vi "Adaptive Parameter 32f.vi"(8 "Error In":errorcluster, 10 "Dynamic Anisotropic Filter Parameters":T1={"Kappa Min"=0.5, "Kappa Max"=10.0, "Time Step"=0.1, "Total Time"=2.0}, 11 "Anisotropic Filter Object":T2={"Device In"=0, "Convolution Object"={"Device In"=0, "Program Handle"=0, "Kernel Memory Object"={"Device ID"=0, "Memeroy ID"=0, "Dimension"={"Depth"=0, "Height"=0, "Width"=0}, "Memory Type"=enum."32f"}, "Convolved Memory Object"={"Device ID"=0, "Memeroy ID"=0, "Dimension"={"Depth"=0, "Height"=0, "Width"=0}, "Memory Type"=enum."32f"}}, "Imag Kernel"=[], "Real Kernel"=[], "Convolved Buffer"={"Device ID"=0, "Memeroy ID"=0, "Dimension"={"Depth"=0, "Height"=0, "Width"=0}, "Memory Type"=enum."32f"}, "Program Handle"=0, "Ansiotropic Filter Parameters"={"Time Step"=0.0, "Total Time"=0.5, "Std. Deviation"=0.0, "Gaussian Filter X Size"=1, "Gaussian Filter Y Size"=1, "Gaussian Filter Z Size"=1}, "Raw Data"={"Device ID"=0, "Memeroy ID"=0, "Dimension"={"Depth"=0, "Height"=0, "Width"=0}, "Memory Type"=enum."32f"}, "Buffer 3"={"Device ID"=0, "Memeroy ID"=0, "Dimension"={"Depth"=0, "Height"=0, "Width"=0}, "Memory Type"=enum."32f"}, "Dimensions"={"Depth"=1, "Height"=1, "Width"=1}} {"Dimensions"."Width" min=1; "Dimensions"."Height" min=1; "Dimensions"."Depth" min=1; "Buffer 3"."Dimension"."Width" min=1; "Buffer 3"."Dimension"."Height" min=1; "Buffer 3"."Dimension"."Depth" min=1; "Raw Data"."Dimension"."Width" min=1; "Raw Data"."Dimension"."Height" min=1; "Raw Data"."Dimension"."Depth" min=1; "Ansiotropic Filter Parameters"."Gaussian Filter Z Size" min=1 max=99 step=2; "Ansiotropic Filter Parameters"."Gaussian Filter Y Size" min=1 max=99 step=2; "Ansiotropic Filter Parameters"."Gaussian Filter X Size" min=1 max=99 step=2; "Convolved Buffer"."Dimension"."Width" min=1; "Convolved Buffer"."Dimension"."Height" min=1; "Convolved Buffer"."Dimension"."Depth" min=1; "Convolution Object"."Convolved Memory Object"."Dimension"."Width" min=1; "Convolution Object"."Convolved Memory Object"."Dimension"."Height" min=1; "Convolution Object"."Convolved Memory Object"."Dimension"."Depth" min=1; "Convolution Object"."Kernel Memory Object"."Dimension"."Width" min=1; "Convolution Object"."Kernel Memory Object"."Dimension"."Height" min=1; "Convolution Object"."Kernel Memory Object"."Dimension"."Depth" min=1}) -> (0 "Error Out":errorcluster, 3 "Anisotropic Filter Object Out":T2={"Device In"=0, "Convolution Object"={"Device In"=0, "Program Handle"=0, "Kernel Memory Object"={"Device ID"=0, "Memeroy ID"=0, "Dimension"={"Depth"=0, "Height"=0, "Width"=0}, "Memory Type"=enum."32f"}, "Convolved Memory Object"={"Device ID"=0, "Memeroy ID"=0, "Dimension"={"Depth"=0, "Height"=0, "Width"=0}, "Memory Type"=enum."32f"}}, "Imag Kernel"=[], "Real Kernel"=[], "Convolved Buffer"={"Device ID"=0, "Memeroy ID"=0, "Dimension"={"Depth"=0, "Height"=0, "Width"=0}, "Memory Type"=enum."32f"}, "Program Handle"=0, "Ansiotropic Filter Parameters"={"Time Step"=0.0, "Total Time"=0.5, "Std. Deviation"=0.0, "Gaussian Filter X Size"=1, "Gaussian Filter Y Size"=1, "Gaussian Filter Z Size"=1}, "Raw Data"={"Device ID"=0, "Memeroy ID"=0, "Dimension"={"Depth"=0, "Height"=0, "Width"=0}, "Memory Type"=enum."32f"}, "Buffer 3"={"Device ID"=0, "Memeroy ID"=0, "Dimension"={"Depth"=0, "Height"=0, "Width"=0}, "Memory Type"=enum."32f"}, "Dimensions"={"Depth"=1, "Height"=1, "Width"=1}} {"Dimensions"."Width" min=1; "Dimensions"."Height" min=1; "Dimensions"."Depth" min=1; "Buffer 3"."Dimension"."Width" min=1; "Buffer 3"."Dimension"."Height" min=1; "Buffer 3"."Dimension"."Depth" min=1; "Raw Data"."Dimension"."Width" min=1; "Raw Data"."Dimension"."Height" min=1; "Raw Data"."Dimension"."Depth" min=1; "Ansiotropic Filter Parameters"."Gaussian Filter Z Size" min=1 max=99 step=2; "Ansiotropic Filter Parameters"."Gaussian Filter Y Size" min=1 max=99 step=2; "Ansiotropic Filter Parameters"."Gaussian Filter X Size" min=1 max=99 step=2; "Convolved Buffer"."Dimension"."Width" min=1; "Convolved Buffer"."Dimension"."Height" min=1; "Convolved Buffer"."Dimension"."Depth" min=1; "Convolution Object"."Convolved Memory Object"."Dimension"."Width" min=1; "Convolution Object"."Convolved Memory Object"."Dimension"."Height" min=1; "Convolution Object"."Convolved Memory Object"."Dimension"."Depth" min=1; "Convolution Object"."Kernel Memory Object"."Dimension"."Width" min=1; "Convolution Object"."Kernel Memory Object"."Dimension"."Height" min=1; "Convolution Object"."Kernel Memory Object"."Dimension"."Depth" min=1}, 4 "Time in ms":dbl)   [LabVIEW 2012, in "OpenCLV x64.lvlib"]
uses:
  OpenCLV x64.lvlib
  Controls/Anisotropic Filter Object.ctl
  Controls/Device ID.ctl
  Controls/Convolution Object.ctl
  Controls/Program Handle.ctl
  Controls/Memory Object.ctl
  Controls/Memory ID.ctl
  User Controls/Array Dimensions.ctl
  Controls/Memory Type.ctl
  Controls/Anisotropic Filter Parameters.ctl
  Read Memory/ReadMemory_32f.vi
  Set Kernel Arguments/Set Kernel Arguments Memory Object.vi
  Set Kernel Arguments/Set Kernel Arguments 32f.vi
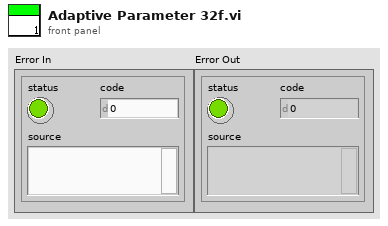
[diagram p1: front panel]
types:
  T1 = cluster{"Kappa Min":sgl, "Kappa Max":sgl, "Time Step":sgl, "Total Time":sgl}
  T2 = typedef "OpenCLV x64.lvlib/Anisotropic Filter Object.ctl" = cluster{"Device In":T3, "Convolution Object":T4, "Imag Kernel":sgl[][][], "Real Kernel":sgl[][][], "Convolved Buffer":T6, "Program Handle":T5, "Ansiotropic Filter Parameters":T10, "Raw Data":T6, "Buffer 3":T6, "Dimensions":T8}
  T3 = typedef "OpenCLV x64.lvlib/Device ID.ctl" = u64
  T4 = typedef "OpenCLV x64.lvlib/Convolution Object.ctl" = cluster{"Device In":T3, "Program Handle":T5, "Kernel Memory Object":T6, "Convolved Memory Object":T6}
  T5 = typedef "OpenCLV x64.lvlib/Program Handle.ctl" = u64
  T6 = typedef "OpenCLV x64.lvlib/Memory Object.ctl" = cluster{"Device ID":T3, "Memeroy ID":T7, "Dimension":T8, "Memory Type":T9}
  T7 = typedef "OpenCLV x64.lvlib/Memory ID.ctl" = u64
  T8 = typedef "Array Dimensions.ctl" = cluster{"Depth":u64, "Height":u64, "Width":u64}
  T9 = typedef "OpenCLV x64.lvlib/Memory Type.ctl" = enum16{"32f", "u8", "i8", "u16", "i16", "u32", "i32", "64f"}
  T10 = typedef "OpenCLV x64.lvlib/Anisotropic Filter Parameters.ctl" = cluster{"Time Step":sgl, "Total Time":sgl, "Std. Deviation":sgl, "Gaussian Filter X Size":u32, "Gaussian Filter Y Size":u32, "Gaussian Filter Z Size":u32}
  T11 = typedef "OpenCLV x64.lvlib/Kernel Handle.ctl" = u64
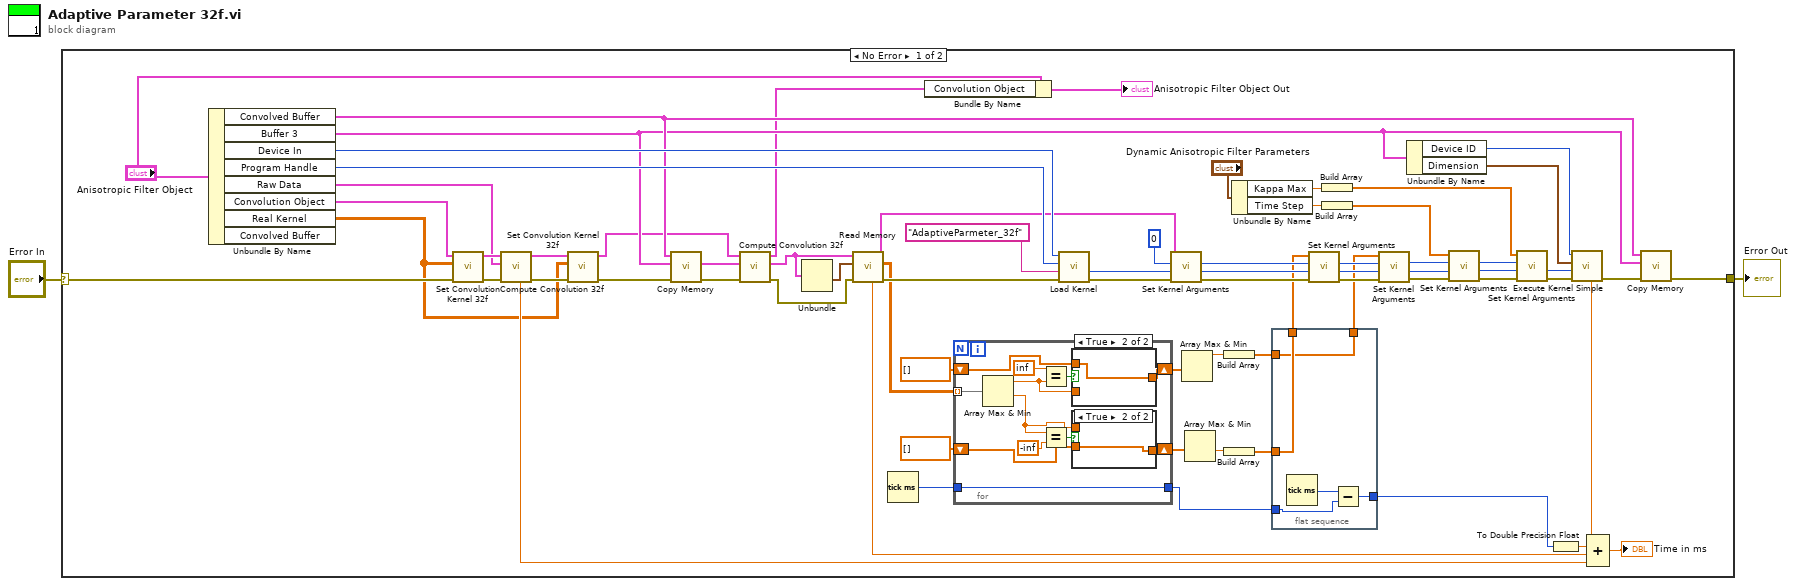
[diagram p0: block diagram]
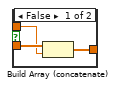
[diagram p2: hidden frame]
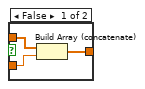
[diagram p3: hidden frame]
diagram:
  n1 = case shown="No Error" "Error In" {
    selector: "Error In" -> [w71 w98]
    tunnel: [w42 w98] -> w1
    frame No Error {
      n2 = Unbundle By Name("Anisotropic Filter Object") -> ("Convolved Buffer"=w25:T6, "Buffer 3"=w24:T6, "Device In"=w66:T3, "Program Handle"=w67:T5, "Raw Data"=w30:T6, "Convolution Object"=w72:T4, "Real Kernel"=w31:sgl[][][])  [unwired: 1 out]
      n3 = call "Set Convolution Kernel 32f.vi"("Error In"=w71, "Kernel In"=w31, "Convolution Object"=w72) -> ("Error Out"=w69:errorcluster, "Convolution Object Out"=w70:T4)  [unwired: 7 in]
      n4 = call "Compute Convolution 32f.vi"("Error In"=w69, "Input Memory"=w30, "Convolution Object"=w70) -> ("Error Out"=w32:errorcluster, "Convolution Object Out"=w29:T4, "Time in ms"=w45:dbl)  [unwired: 5 in, 1 out]
      n5 = call "Set Convolution Kernel 32f.vi"("Error In"=w32, "Kernel In"=w31, "Convolution Object"=w29) -> ("Error Out"=w28:errorcluster, "Convolution Object Out"=w23:T4)  [unwired: 7 in]
      n6 = call "Copy Memory.vi"("Error In"=w28, "Destination Object"=w24, "Source Object"=w25) -> ("Error Out"=w27:errorcluster, "Destination Object Out"=w26:T6)  [unwired: 6 in, 1 out]
      n7 = call "Compute Convolution 32f.vi"("Error In"=w27, "Input Memory"=w26, "Convolution Object"=w23) -> ("Error Out"=w22:errorcluster, "Convolved Memory"=w4:T6, "Convolution Object Out"=w21:T4)  [unwired: 5 in, 1 out]
      n8 = Unbundle(w4) -> ("Dimension"=w3:T8)  [unwired: 3 out]
      n9 = call-poly "Read Memory.vi"("Error In"=w22, "Dimensions"=w3, "Memory Object In"=w4) -> ("Error Out"=w68:errorcluster, "Data Out"=w37:sgl[][][], "Memory Object Out"=w61:T6, "ms"=w46:dbl)  [unwired: 5 in]
      n10 = Tick Count (ms)() -> (millisecond timer value=w11:u32)
      n11 = Bundle By Name(cluster="Anisotropic Filter Object", "Convolution Object"=w21) -> (→"Anisotropic Filter Object Out":T2)
      n12 = for {
        tunnel: w37 -> [w89] mode=indexing
        shift-right: [w82] -> w15
        shift-left: sgl[] [] -> [w81]
        shift-right: [w80] -> w14
        shift-left: sgl[] [] -> [w79]
        tunnel: w11 -> [w78]
        tunnel: [w78] -> w6
        n13 = Array Max & Min(array=w89) -> (max value=w83:sgl, min value=w84:sgl)  [unwired: 2 out]
        n14 = Equal?(x=inf, y=w83) -> (x = y?=w85:bool)
        n15 = Equal?(x=w84, y=-inf) -> (x = y?=w87:bool)
        n16 = case shown="True" w85 {
          tunnel: w83 -> [w96 _]
          tunnel: [w95 w97] -> w82
          tunnel: w81 -> [w94 w97]
          frame False {
            n17 = Build Array (concatenate)(w94, w96) -> (w95:sgl[])
          }
          frame True {
          }
        }
        n18 = case shown="True" w87 {
          tunnel: w84 -> [w91 _]
          tunnel: w79 -> [w92 w93]
          tunnel: [w90 w93] -> w80
          frame False {
            n19 = Build Array (concatenate)(w92, w91) -> (w90:sgl[])
          }
          frame True {
          }
        }
      }
      n20 = call "Load Kernel.vi"("Error In"=w68, "Kernel Name"="AdaptiveParmeter_32f", "Program Handle"=w67, "Device In"=w66) -> ("Error Out"=w64:errorcluster, "Kernel Handle"=w63:T11)  [unwired: 4 in, 2 out]
      n21 = call-poly "Set Kernel Arguments.vi"("Error In"=w64, "Kernel Handle"=w63, "Argument Number"=0, "Memory Object"=w61) -> ("Error Out"=w60:errorcluster, "Kernel Handle out"=w59:T11, "Auto Inc Arugment Number"=w58:i32)  [unwired: 5 in]
      n22 = Array Max & Min(array=w15) -> (max value=w13:sgl)  [unwired: 3 out]
      n23 = Array Max & Min(array=w14) -> (min value=w12:sgl)  [unwired: 3 out]
      n24 = Build Array(w13) -> (w7:sgl[])
      n25 = Build Array(w12) -> (w10:sgl[])
      n26 = Unbundle By Name("Dynamic Anisotropic Filter Parameters") -> ("Kappa Max"=w19:sgl, "Time Step"=w18:sgl)
      n27 = flat-sequence {
        tunnel: [w76] -> w9
        tunnel: w10 -> [w76]
        tunnel: [w75] -> w8
        tunnel: w7 -> [w75]
        tunnel: w6 -> [w74]
        tunnel: [w73] -> w5
        frame #0 {
          n28 = Tick Count (ms)() -> (millisecond timer value=w77:u32)
          n29 = Subtract(x=w77, y=w74) -> (x-y=w73:u32)
        }
      }
      n30 = call-poly "Set Kernel Arguments.vi"("Error In"=w60, "Kernel Handle"=w59, "Argument Number"=w58, "32f Constant"=w9) -> ("Error Out"=w55:errorcluster, "Kernel Handle out"=w56:T11, "Auto Inc Arugment Number"=w57:i32)  [unwired: 5 in]
      n31 = Build Array(w19) -> (w53:sgl[])
      n32 = Build Array(w18) -> (w54:sgl[])
      n33 = call-poly "Set Kernel Arguments.vi"("Error In"=w55, "Kernel Handle"=w56, "Argument Number"=w57, "32f Constant"=w8) -> ("Error Out"=w51:errorcluster, "Kernel Handle out"=w50:T11, "Auto Inc Arugment Number"=w49:i32)  [unwired: 5 in]
      n34 = Unbundle By Name(w24) -> ("Device ID"=w39:T3, "Dimension"=w35:T8)
      n35 = call-poly "Set Kernel Arguments.vi"("Error In"=w51, "Kernel Handle"=w50, "Argument Number"=w49, "32f Constant"=w54) -> ("Error Out"=w52:errorcluster, "Kernel Handle out"=w48:T11, "Auto Inc Arugment Number"=w47:i32)  [unwired: 5 in]
      n36 = call-poly "Set Kernel Arguments.vi"("Error In"=w52, "Kernel Handle"=w48, "Argument Number"=w47, "32f Constant"=w53) -> ("Error Out"=w41:errorcluster, "Kernel Handle out"=w40:T11)  [unwired: 5 in, 1 out]
      n37 = To Double Precision Float(number=w5) -> (double precision float=w44:dbl)
      n38 = call "Execute Kernel Simple.vi"("Error In"=w41, "Kernel Handle"=w40, "Thread Dimensions"=w35, "Device In"=w39) -> ("Error Out"=w36:errorcluster, "Time in ms"=w38:dbl)  [unwired: 4 in, 2 out]
      n39 = Compound Arithmetic op=ADD(w38, w44, w46, w45) -> (→"Time in ms":dbl)
      n40 = call "Copy Memory.vi"("Error In"=w36, "Destination Object"=w24, "Source Object"=w25) -> ("Error Out"=w42:errorcluster)  [unwired: 6 in, 2 out]
    }
    frame Error {
    }
  }
  "Error Out" <- w1
